vi "Set Scroll bar State.vi"(8 "error in (no error)":errorcluster, 10 "Horizontal Scrollbar Visibility":T1(ring), 11 "Ref Pane in":refnum<vi>) -> (0 "error out":errorcluster, 3 "Ref Pane Out":refnum<vi>)   [LabVIEW 2017]
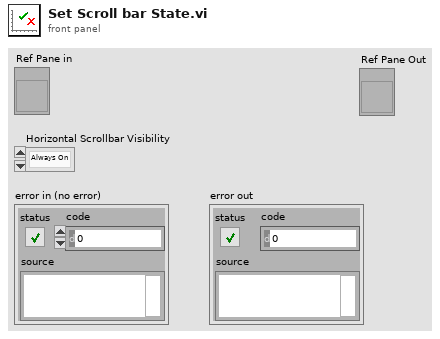
[diagram p1: front panel]
types:
  T1 = enum16{"Always On", "Always Off", "Off While Running"}
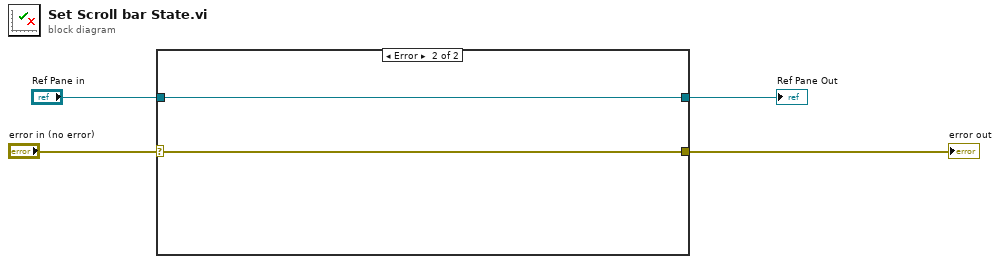
[diagram p0: block diagram]
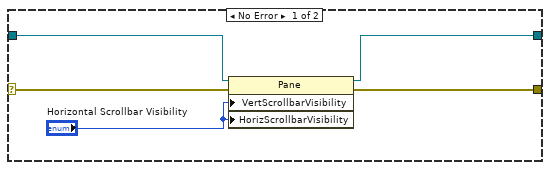
[diagram p2: hidden frame]
diagram:
  n1 = case shown="Error" "error in (no error)" {
    selector: "error in (no error)" -> [w7 w11]
    tunnel: [w8 w11] -> w4
    tunnel: "Ref Pane in" -> [w6 w10]
    tunnel: [w5 w10] -> w1
    frame No Error {
      n2 = property on="Property Node" class="Pane"(reference=w6, error in=w7, "VertScrollbarVisibility"="Horizontal Scrollbar Visibility", "HorizScrollbarVisibility"="Horizontal Scrollbar Visibility") -> (reference out=w5:refnum<vi>, error out=w8:errorcluster)
    }
    frame Error {
    }
  }
  "error out" <- w4
  "Ref Pane Out" <- w1
